vi "Publish.vi"(8 "error in (no error)":errorcluster, 11 "Mediator in":refnum<class "Mediator.lvclass">) -> (0 "error out":errorcluster, 3 "Mediator out":refnum<class "Mediator.lvclass">)   [LabVIEW 2015, in "Mediator.lvlib" / "Mediator.lvclass"]
uses:
  Mediator.lvclass
  Mediator.lvclass/Mediator.ctl
  Topic Messages/Notify Subscribers Msg/Notify Subscribers Msg.lvclass/Notify Subscribers Msg.ctl
  <vilib>/ActorFramework/Message Enqueuer/Message Enqueuer.lvclass/Message Enqueuer.ctl
  <vilib>/ActorFramework/Message Enqueuer/Enqueue.vi
  <vilib>/ActorFramework/Message Priority Queue/Priority Enqueue.vi
  Topic Messages/Notify Subscribers Msg/Notify Subscribers Msg.lvclass
  TopicLookupTable/TopicLookupTable.lvclass
  Topic/Topic.lvclass
  <vilib>/ActorFramework/Actor/Actor.lvclass
panel:
  in  "Topic Name":string
  in  "Data to Publish":variant
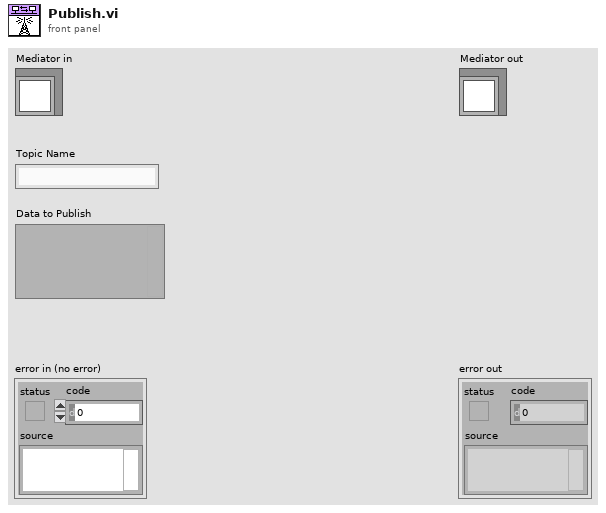
[diagram p1: front panel]
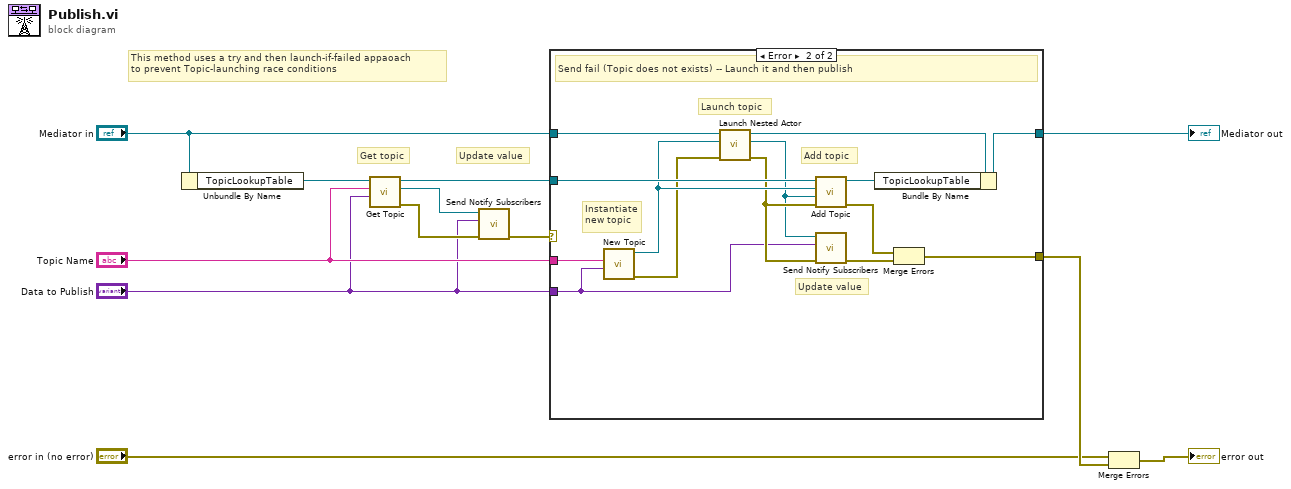
[diagram p0: block diagram]
diagram:
  # "This method uses a try and then launch-if-failed appaoach\nto prevent Topic-launching race conditions"
  # "Update value"
  # "Get topic"
  n1 = Unbundle By Name("Mediator in") -> ("TopicLookupTable"=w11:refnum<class "TopicLookupTable.lvclass">)
  n2 = call "Get Topic.vi"("Topic Type"="Data to Publish", "Topic Name"="Topic Name", "TopicLookupTable in"=w11) -> ("error out"=w7:errorcluster, "Topic Refnum"=w12:refnum<class "Message Enqueuer.lvclass">, "TopicLookupTable out"=w10:refnum<class "TopicLookupTable.lvclass">)  [unwired: 5 in, 1 out]
  n3 = call "Send Notify Subscribers.vi"("error in (no error)"=w7, "Topic Data"="Data to Publish", "Message Enqueuer"=w12) -> ("error out"=w9:errorcluster)  [unwired: 7 in, 1 out]
  n4 = case shown="Error" w9 {
    selector: w9 -> [w13 _]
    tunnel: w10 -> [_ w24]
    tunnel: "Mediator in" -> [w14 w28]
    tunnel: [w14 w27] -> w5
    tunnel: "Topic Name" -> [_ w25]
    tunnel: "Data to Publish" -> [_ w15]
    tunnel: [w13 w18] -> w8
    frame No Error {
      # "Subscribe OK (Topic is alive)"
    }
    frame Error {
      # "Launch topic"
      # "Add topic"
      # "Update value"
      # "Instantiate\nnew topic"
      # "Send fail (Topic does not exists) -- Launch it and then publish"
      n5 = call "New Topic.vi"("Data Type"=w15, "Name"=w25) -> ("error out"=w21:errorcluster, "Topic out"=w22:refnum<class "Topic.lvclass">)  [unwired: 8 in]
      n6 = call <vilib>:"Launch Nested Actor.vi"("error in (no error)"=w21, "Nested Actor"=w22, "Caller Actor in"=w28) -> ("error out"=w17:errorcluster, "Nested Actor's Enqueuer"=w16:refnum<class "Message Enqueuer.lvclass">, "Caller Actor out"=w26:refnum<class "Mediator.lvclass">)  [unwired: 6 in]
      n7 = call "Add Topic.vi"("error in (no error)"=w17, "Topic Enqueuer"=w16, "Topic Object"=w22, "TopicLookupTable in"=w24) -> ("error out"=w20:errorcluster, "TopicLookupTable out"=w23:refnum<class "TopicLookupTable.lvclass">)  [unwired: 5 in, 1 out]
      n8 = call "Send Notify Subscribers.vi"("error in (no error)"=w17, "Topic Data"=w15, "Message Enqueuer"=w16) -> ("error out"=w19:errorcluster)  [unwired: 7 in, 1 out]
      n9 = Bundle By Name(cluster=w26, "TopicLookupTable"=w23) -> (w27:refnum<class "Mediator.lvclass">)
      n10 = Merge Errors(w20, w19) -> (w18:errorcluster)
    }
  }
  "Mediator out" <- w5
  n11 = Merge Errors("error in (no error)", w8) -> (→"error out":errorcluster)
